vi "Ryans Project Properties.vi"   [LabVIEW 2019]
doc: "Launches the <b>Tools > Project Properties...</b> dialog.\n\nCreated by: Ryan Pacini"
types:
  T1 = enum32{"Bad", "Idle", "Run top level", "Running"}
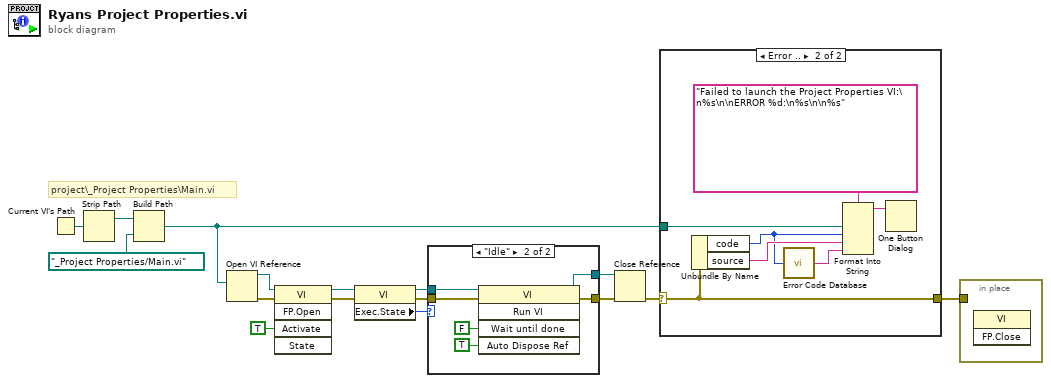
[diagram p0: block diagram]
diagram:
  # "project\\_Project Properties\\Main.vi"
  n1 = Current VI's Path() -> (path=w16:path)
  n2 = Strip Path(path=w16) -> (stripped path=w15:path)  [unwired: 1 out]
  n3 = Build Path(base path=w15, name or relative path=path "_Project Properties/Main.vi") -> (appended path=w2:path)
  n4 = Open VI Reference(vi path=w2) -> (vi reference=w11:refnum<vi>, error out=w14:errorcluster)  [unwired: 5 in]
  n5 = invoke class="VI" method="FP.Open"(reference=w11, error in=w14, "Activate"=TRUE ("Activate?")) -> (reference out=w10:refnum<vi>, error out=w7:errorcluster)  [unwired: 2 in, 3 out]
  n6 = property class="VI"(reference=w10, error in=w7) -> (reference out=w8:refnum<vi>, error out=w6:errorcluster, "Exec.State"=w5:T1)
  n7 = case shown="\"Idle\"" w5 {
    tunnel: [w17 w22] -> w13
    tunnel: [w18 w21] -> w12
    tunnel: w8 -> [w18 w20]
    tunnel: w6 -> [w17 w19]
    frame "Bad", "Run top level", "Running" {
      # "Already running"
    }
    frame "Idle" {
      n8 = invoke class="VI" method="Run VI"(reference=w20, error in=w19, "Wait until done"=FALSE ("Wait Until Done"), "Auto Dispose Ref"=TRUE ("Auto Dispose Reference")) -> (reference out=w21:refnum<vi>, error out=w22:errorcluster)  [unwired: 1 in, 3 out]
    }
  }
  n9 = Close Reference(reference=w12, error in (no error)=w13) -> (error out=w3:errorcluster)
  n10 = case shown="Error .." w3 {
    selector: w3 -> [w25 w28]
    tunnel: w2 -> [_ w29]
    tunnel: [w25 w28] -> w1
    frame No Error {
    }
    frame Error {
      n11 = Unbundle By Name(w28) -> ("code"=w27:i32, "source"=w32:string)
      n12 = call <vilib>:"Error Code Database.vi"("Error Code"=w27) -> ("Error Text"=w26:string)
      n13 = Format Into String(format string="Failed to launch the Project Properties VI:\n%s\n\nERROR %d:\n%s\n\n%s", w29, w27, w32, w26) -> (resulting string=w30:string)  [unwired: 2 in, 1 out]
      n14 = One Button Dialog(message=w30) -> ()  [unwired: 1 in, 1 out]
    }
  }
  n15 = in-place {
    in-place-border: w1 -> [_]
    n16 = invoke class="VI" method="FP.Close"() -> ()  [unwired: 3 in, 3 out]
  }
